vi "Material Theme Editor.vi"() -> ()   [LabVIEW 2021]
doc: "Convert existing material3 json files exported from Google to be used with TSC Material application VIs.\n\n<b>Code Developed By:</b>\nDaniel Coons\nTechnology Service Corporation\nwww.tsc.com/atcs"
uses:
  Material-Palette/Material-Palette.lvclass
  Material Theme/Material Theme.lvclass
  Material-Scheme/Material-Scheme.lvclass
  user32.dll
  <vilib>/Utility/traverseref.llb/VI Scripting - Traverse.lvlib
  <vilib>/Utility/traverseref.llb/TRef TravTarget.ctl
  Material-Scheme/View-User Colors.vi
  _theme-editor/Theme Config/Theme Config.lvclass
panel:
  in  "palette":bool
  in  "File Interaction":enum32{"convert--buton", "load--buton"}(radio)
  in  "tabs":enum32{"color", "palette", "json", "buttons"}(radio)
  in  "preview":bool
  in  "close":bool
  out "header":bool
  in  "save":bool
  in  "Theme Mode":u16(ring) items=["Light Theme", "Light Medium Contrast", "Light High Contrast", "Dark Theme", "Dark Medium Contrast", "Dark High Constrast"]
  in  "Tab Control":T1(tab)
  out "material JSON output":string
  in  "Color Level":u16(ring) items=["Primary", "Secondary", "Tertiary", "Error", "Primary Fixed", "Secondary Fixed", "Tertiary Fixed"]
  in  "Tab Control file":enum32{"convert", "load"}(tab)
  in  "LabVIEW material theme":path
  in  "json file path":path caption="Material Theme JSON File"
  # "Load a TSC Material Theme legacy XML file to see modes\nand palette colors and convert to JSON format for long-term\nsupport."
  # "Load a JSON M3 theme file from Google to \nview and edit the scheme."
  # "Can be generated through Figma or at:   https://material-foundation.github.io/material-theme-builder/<Material Website>"
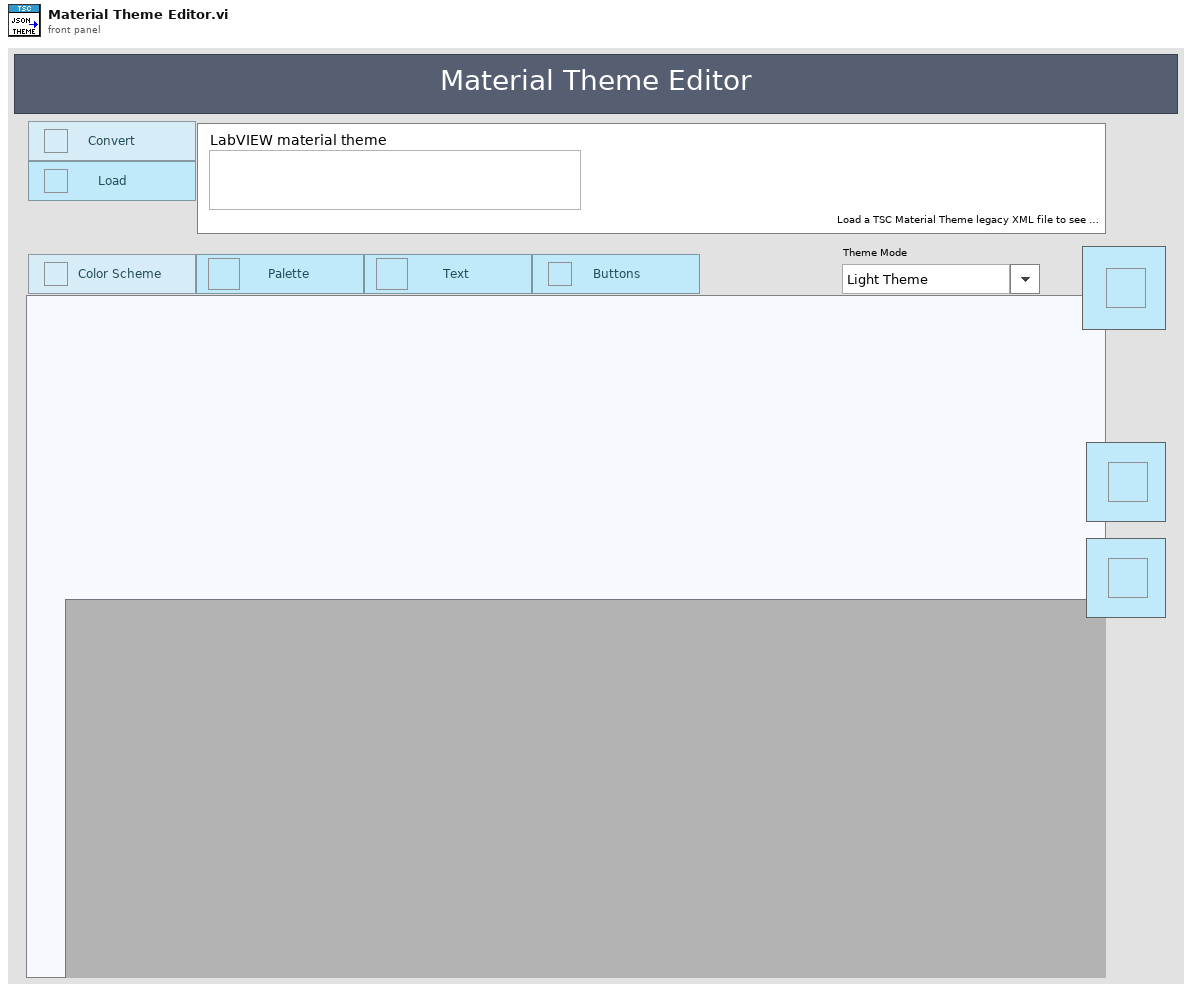
[diagram p1: front panel]
types:
  T1 = enum32{"Color Scheme", "Palette Variations", "JSON String", "buttons"}
  T2 = typedef "TRef TravTarget.ctl" = enum16{"FP", "BD", "Other"}
  T3 = enum16{"open", "replace", "create", "open or create", "replace or create", "replace or create with confirmation"}
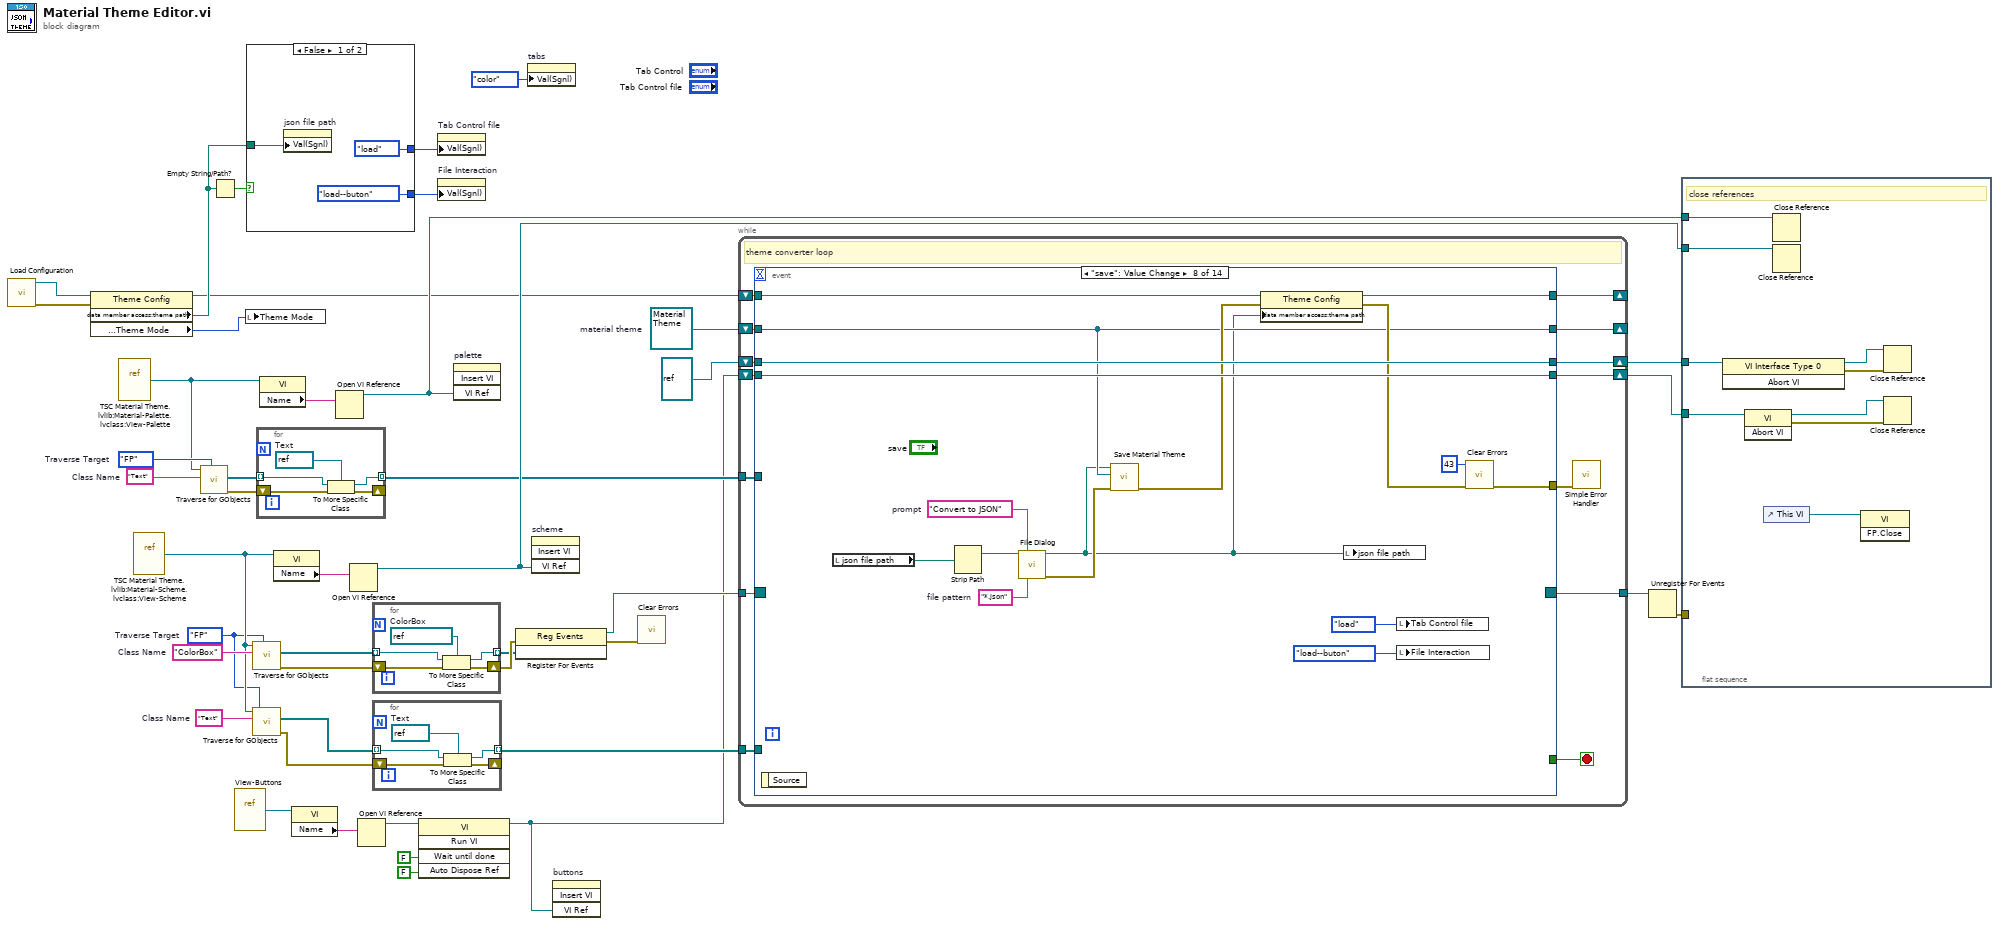
[diagram p0: block diagram]
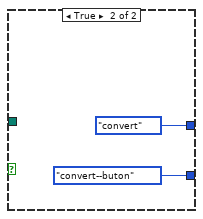
[diagram p2: hidden frame]
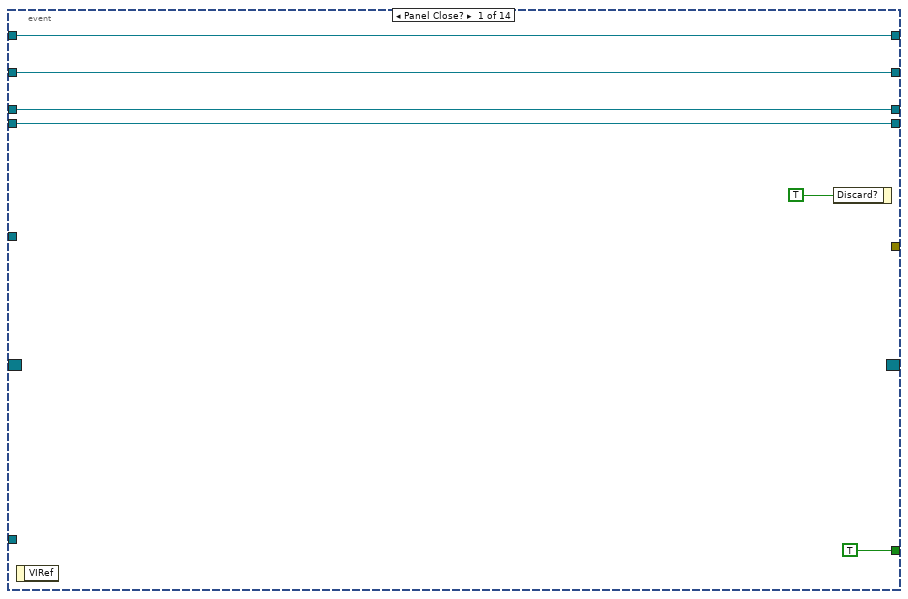
[diagram p3: hidden frame]
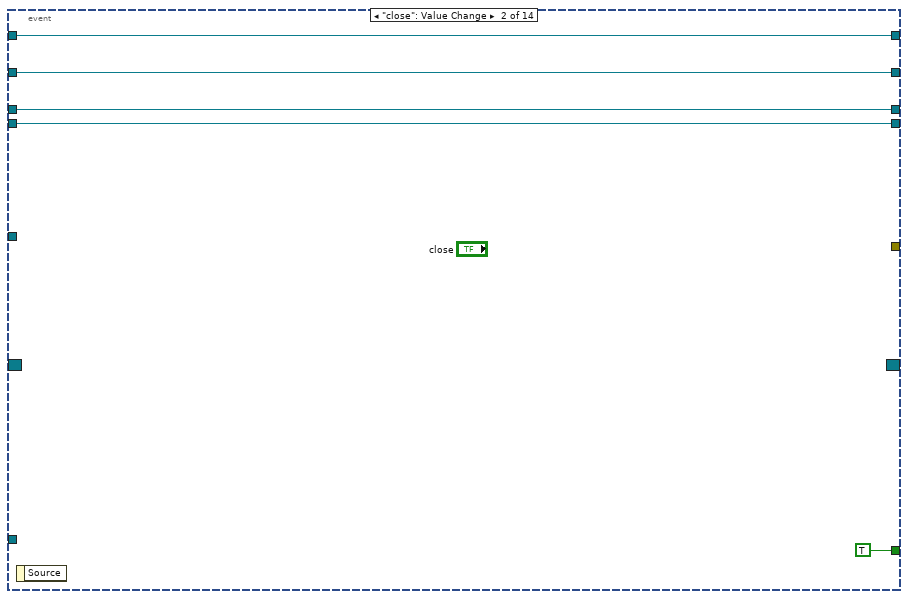
[diagram p4: hidden frame]
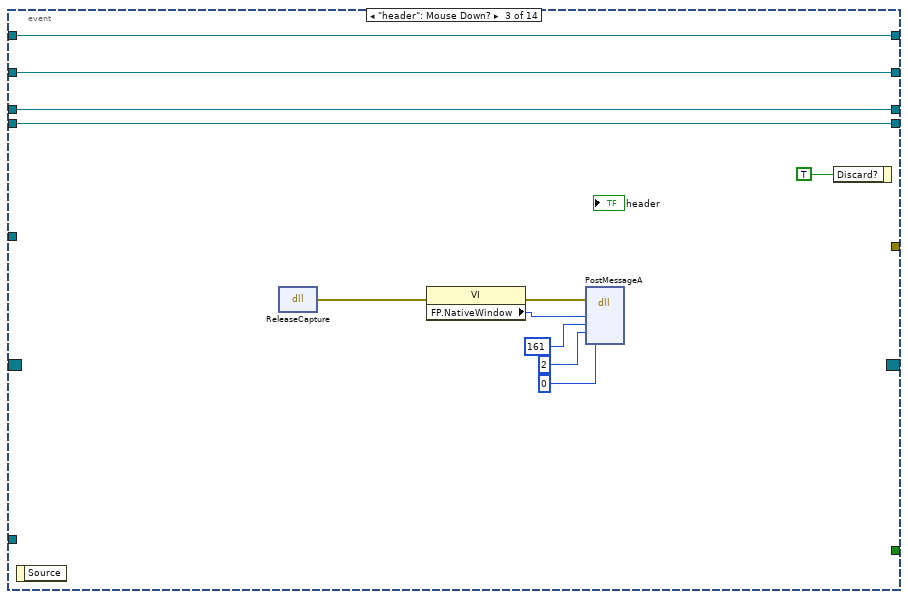
[diagram p5: hidden frame]
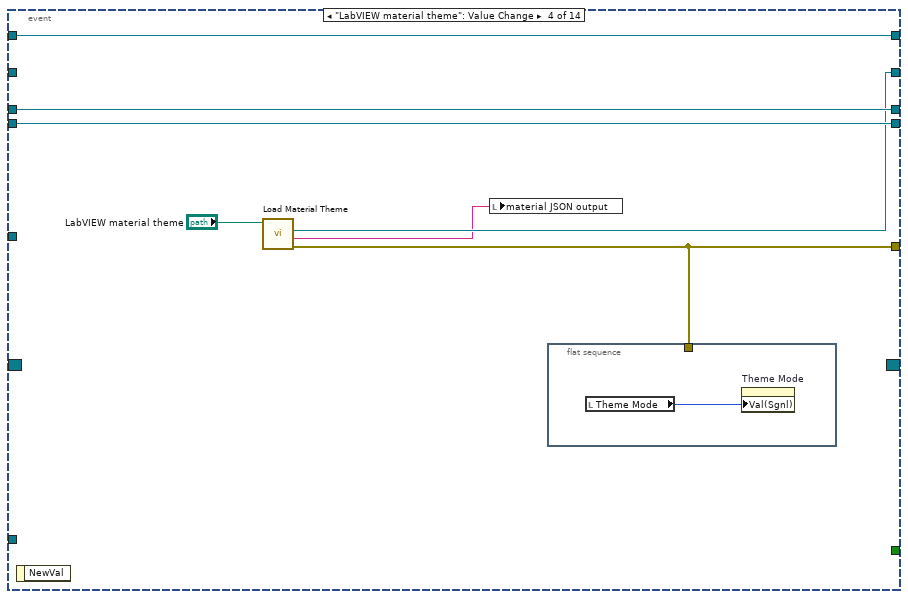
[diagram p6: hidden frame]
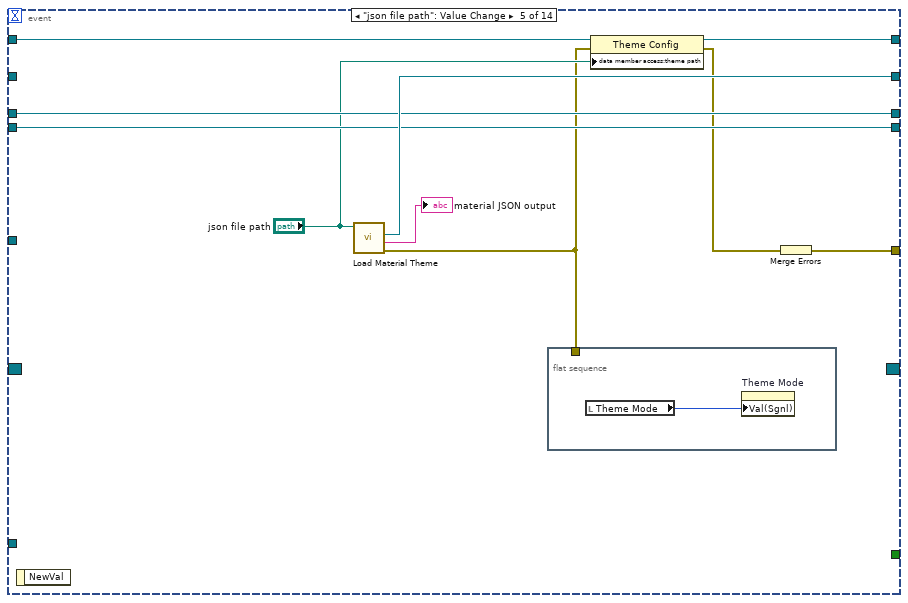
[diagram p7: hidden frame]
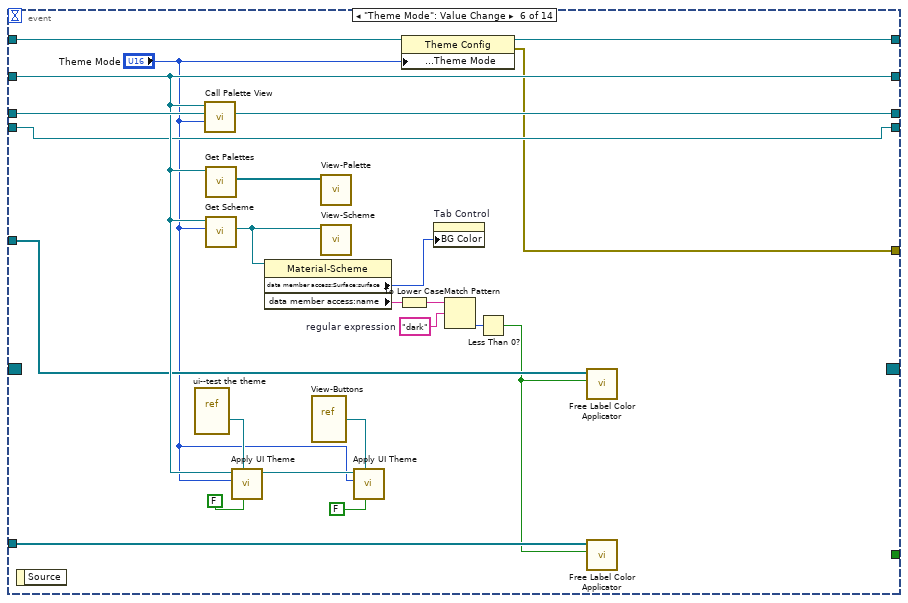
[diagram p8: hidden frame]
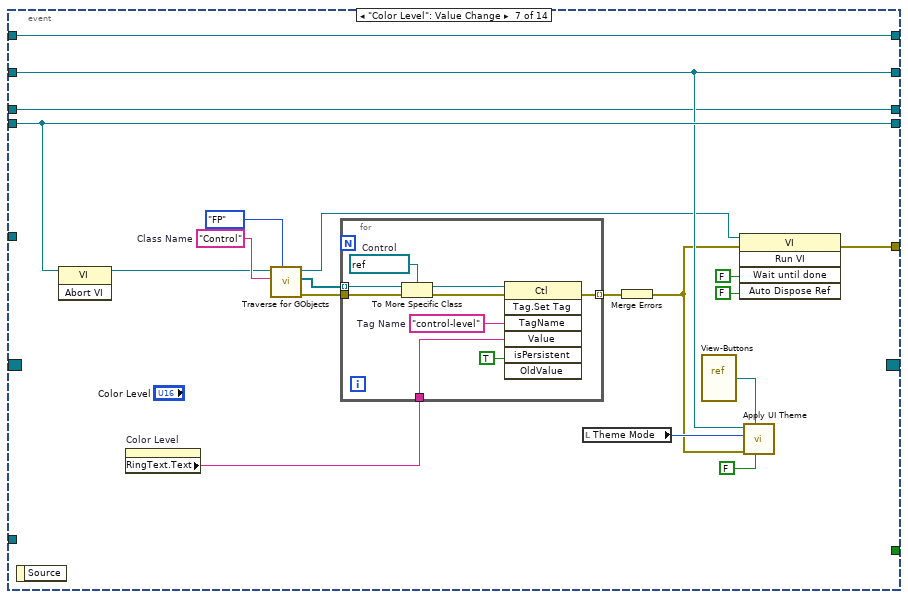
[diagram p9: hidden frame]
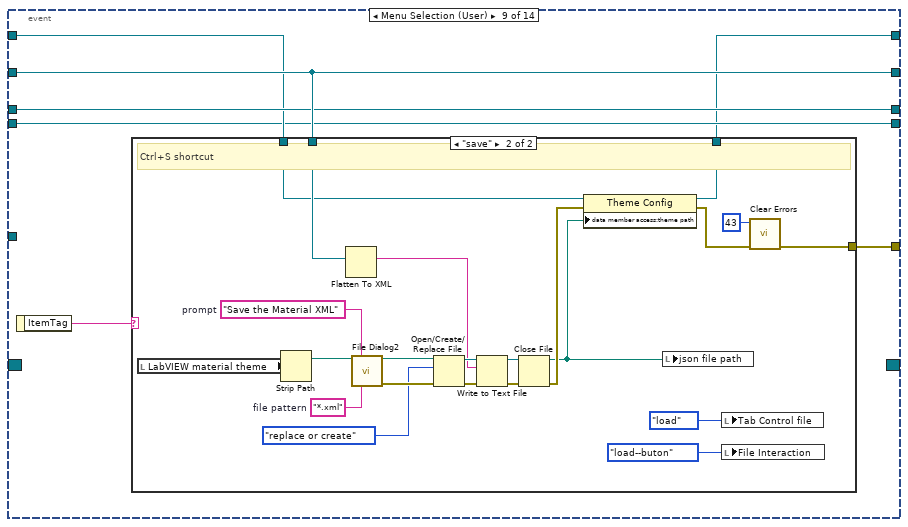
[diagram p10: hidden frame]
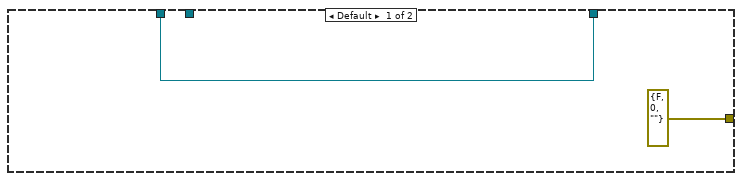
[diagram p11: hidden frame]
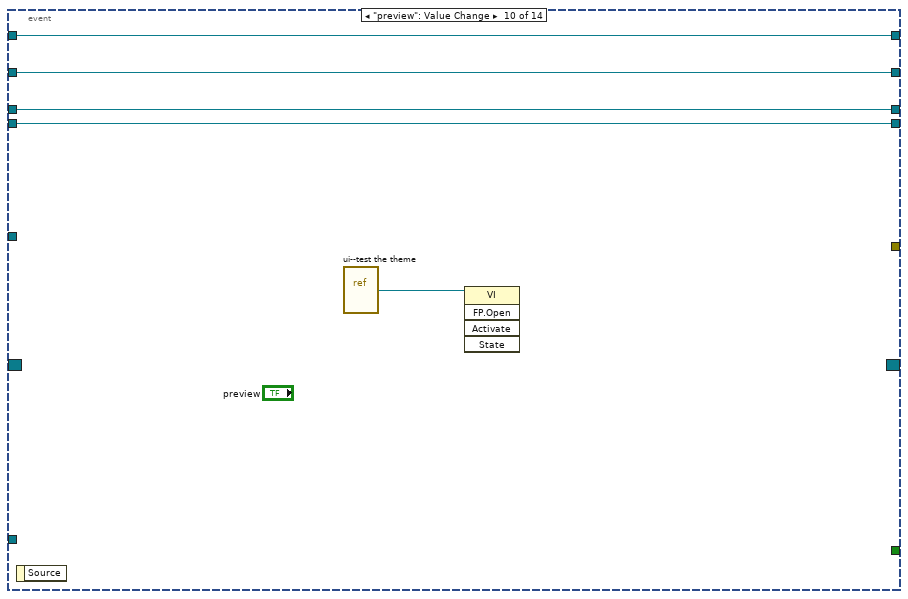
[diagram p12: hidden frame]
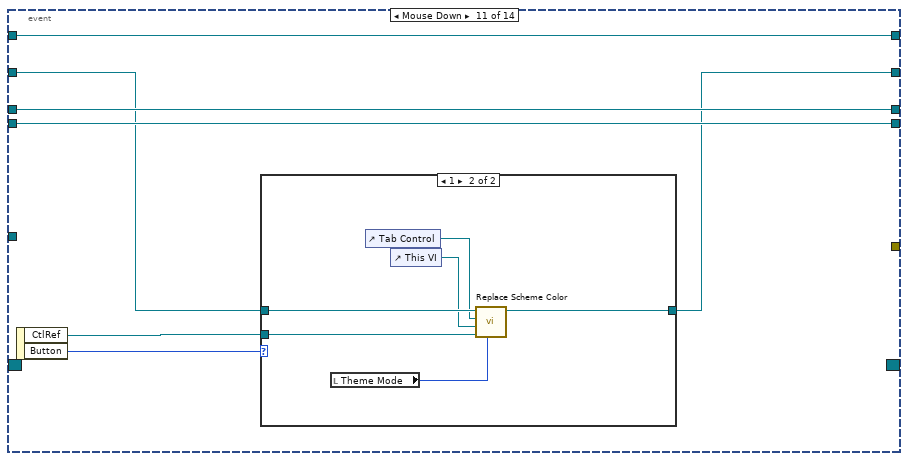
[diagram p13: hidden frame]
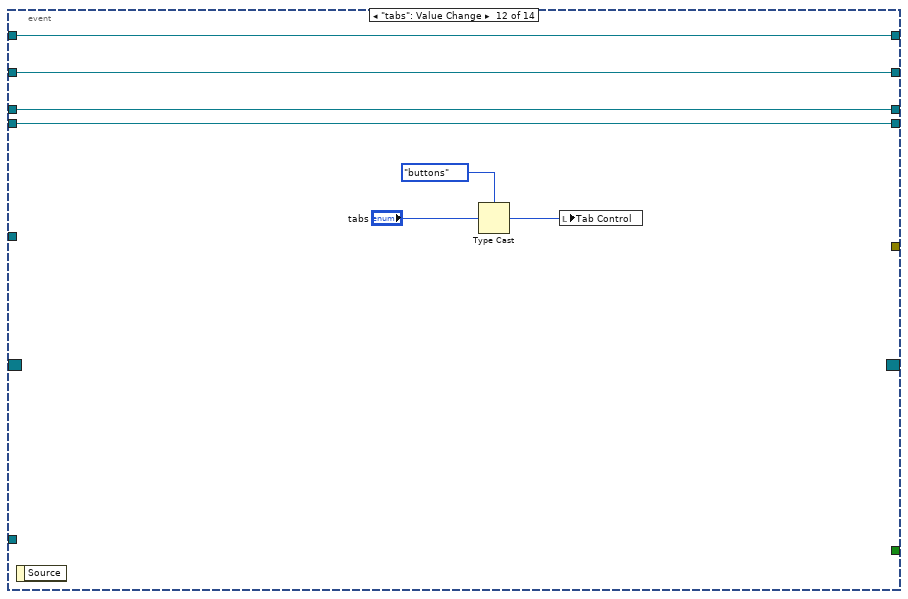
[diagram p15: hidden frame]
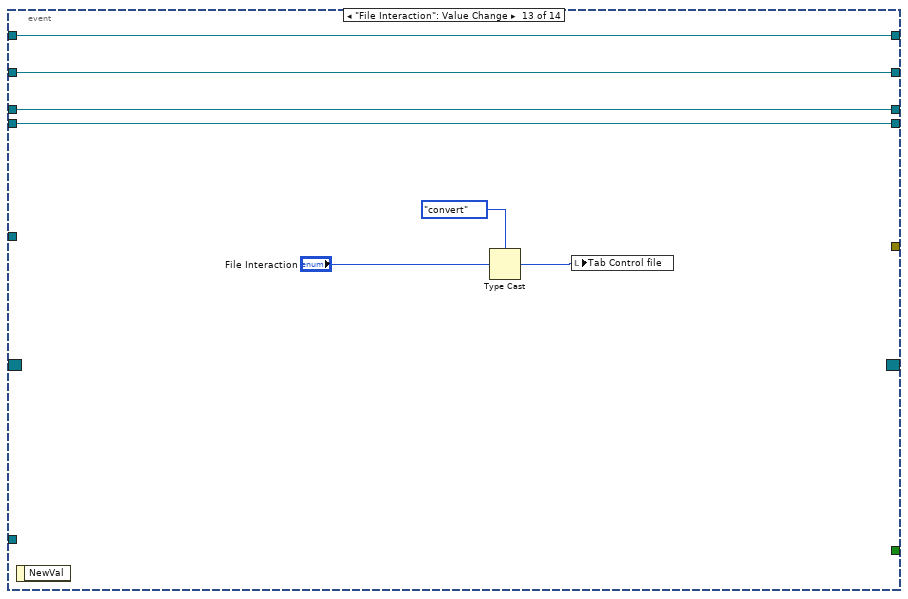
[diagram p16: hidden frame]
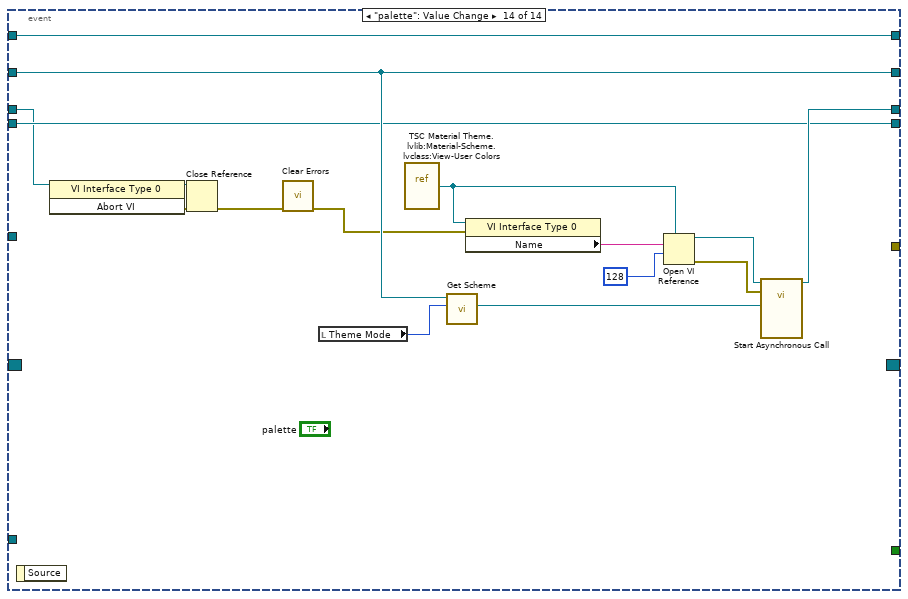
[diagram p17: hidden frame]
diagram:
  w24 = "Text"  # Class Name
  w27 = "Text"  # Class Name
  w28 = TRef_TravTarget."FP"  # Traverse Target
  w30 = refnum<class "Material Theme.lvclass"> refnum  # material theme
  w36 = "ColorBox"  # Class Name
  w22 = TRef_TravTarget."FP"  # Traverse Target
  n1 = call "Load Configuration.vi"() -> ("error out"=w10:errorcluster, "Theme Config out"=w9:refnum<class "Theme Config.lvclass">)  [unwired: 10 in]
  n2 = property class="Theme Config"(reference=w9, error in=w10) -> (reference out=w6:refnum<class "Theme Config.lvclass">, "data member access:theme path"=w8:path, "data member access:Theme Mode"=w3:u16)  [unwired: 1 out]
  n3 = vi-ref "TSC Material Theme.lvlib:Material-Palette.lvclass:View-Palette.vi"() -> (w7:refnum<vi>)
  n4 = vi-ref "TSC Material Theme.lvlib:Material-Scheme.lvclass:View-Scheme.vi"() -> (w23:refnum<vi>)
  n5 = call <vilib>:"Traverse for GObjects.vi"("Traverse Target"=w28, "Class Name"=w27, "VI Refnum"=w7) -> ("error out"=w41:errorcluster, "References"=w26:refnum<vi>[])  [unwired: 5 in, 2 out]
  n6 = Empty String/Path?(string/path=w8) -> (empty?=w29:bool)
  n7 = vi-ref "View-Buttons.vi"() -> (w17:refnum<vi>)
  n8 = local write "Theme Mode"(w3) -> ()
  n9 = case shown="False" w29 {
    tunnel: w8 -> [w47 _]
    tunnel: [enum32{"convert", "load"}."load" ("Value (Signaling)") enum32{"convert", "load"}."convert" ("Value (Signaling)")] -> w2
    tunnel: [enum32{"convert--buton", "load--buton"}."load--buton" ("Value (Signaling)") enum32{"convert--buton", "load--buton"}."convert--buton" ("Value (Signaling)")] -> w1
    frame False {
      n10 = property on="json file path" class="Path"("Val(Sgnl)"=w47) -> ()  [unwired: 2 in, 2 out]
    }
    frame True {
    }
  }
  n11 = call <vilib>:"Traverse for GObjects.vi"("Traverse Target"=w22, "Class Name"=w36, "VI Refnum"=w23) -> ("error out"=w44:errorcluster, "References"=w34:refnum<vi>[])  [unwired: 5 in, 2 out]
  n12 = call <vilib>:"Traverse for GObjects.vi"("Traverse Target"=w22, "Class Name"=w24, "VI Refnum"=w23) -> ("error out"=w40:errorcluster, "References"=w21:refnum<vi>[])  [unwired: 5 in, 2 out]
  n13 = for {
    tunnel: w26 -> [w51] mode=indexing
    shift-right: [w53] -> _
    shift-left: w41 -> [w54]
    tunnel: [w50] -> w25 mode=indexing
    w52 = refnum<vi> refnum  # Text
    n14 = To More Specific Class(target class=w52, reference=w51, error in=w54) -> (specific class reference=w50:refnum<vi>, error out=w53:errorcluster)
  }
  n15 = property class="VI"(reference=w7) -> ("Name"=w39:string)  [unwired: 1 in, 2 out]
  n16 = property class="VI"(reference=w23) -> ("Name"=w38:string)  [unwired: 1 in, 2 out]
  n17 = property class="VI"(reference=w17) -> ("Name"=w16:string)  [unwired: 1 in, 2 out]
  n18 = Open VI Reference(vi path=w39) -> (vi reference=w37:refnum<vi>)  [unwired: 5 in, 1 out]
  n19 = Open VI Reference(vi path=w38) -> (vi reference=w33:refnum<vi>)  [unwired: 5 in, 1 out]
  n20 = Open VI Reference(vi path=w16) -> (vi reference=w18:refnum<vi>)  [unwired: 5 in, 1 out]
  n21 = for {
    tunnel: w34 -> [w56] mode=indexing
    shift-right: [w58] -> w43
    shift-left: w44 -> [w59]
    tunnel: [w55] -> w32 mode=indexing
    w57 = refnum<vi> refnum  # ColorBox
    n22 = To More Specific Class(target class=w57, reference=w56, error in=w59) -> (specific class reference=w55:refnum<vi>, error out=w58:errorcluster)
  }
  n23 = for {
    tunnel: w21 -> [w61] mode=indexing
    shift-right: [w63] -> _
    shift-left: w40 -> [w64]
    tunnel: [w60] -> w20 mode=indexing
    w62 = refnum<vi> refnum  # Text
    n24 = To More Specific Class(target class=w62, reference=w61, error in=w64) -> (specific class reference=w60:refnum<vi>, error out=w63:errorcluster)
  }
  n25 = invoke class="VI" method="Run VI"(reference=w18, "Wait until done"=FALSE ("Wait Until Done"), "Auto Dispose Ref"=FALSE ("Auto Dispose Reference")) -> (reference out=w13:refnum<vi>)  [unwired: 2 in, 4 out]
  n26 = property on="Tab Control file" class="TabCtl (strict)"("Val(Sgnl)"=w2) -> ()  [unwired: 2 in, 2 out]
  n27 = property on="File Interaction" class="RadioBtnsControl (strict)"("Val(Sgnl)"=w1) -> ()  [unwired: 2 in, 2 out]
  n28 = invoke on="palette" class="SubPnl" method="Insert VI"("VI Ref"=w37) -> ()  [unwired: 3 in, 4 out]
  n29 = register-events(error in=w43, w32) -> (reference out=w35:refnum<event-registration>, error out=w42:errorcluster)  [unwired: 1 in]
  n30 = property on="tabs" class="RadioBtnsControl (strict)"("Val(Sgnl)"=enum32{"color", "palette", "json", "buttons"}."color" ("Value (Signaling)")) -> ()  [unwired: 2 in, 2 out]
  n31 = invoke on="scheme" class="SubPnl" method="Insert VI"("VI Ref"=w33) -> ()  [unwired: 3 in, 4 out]
  n32 = invoke on="buttons" class="SubPnl" method="Insert VI"("VI Ref"=w13) -> ()  [unwired: 3 in, 4 out]
  n33 = call <vilib>:"Clear Errors.vi"("error in (no error)"=w42) -> ()  [unwired: 5 in, 2 out]
  n34 = while {
    shift-right: [w76] -> _
    shift-left: w30 -> [w75]
    tunnel: w35 -> [w74]
    tunnel: [w73] -> w31
    tunnel: w25 -> [w72]
    tunnel: w20 -> [w71]
    shift-right: [w69] -> w12
    shift-left: refnum<vi> refnum -> [w68]
    shift-right: [w66] -> _
    shift-left: w6 -> [w67]
    shift-right: [w65] -> w4
    shift-left: w13 -> [w70]
    stop <- w77 stop-if-true
    # "theme converter loop"
    n35 = event shown="[7] \"save\": Value Change" {
      selector: w74 -> [_ _ _ _ _ _ _ _ _ _ _ _ _ _]
      dyn-events: [_ _ _ _ _ _ _ _ _ _ _ _ _ _] -> w73
      timeout: _ -> [_ _ _ _ _ _ _ _ _ _ _ _ _ _]
      tunnel: [TRUE TRUE _ _ _ _ _ _ _ _ _ _ _ _] -> w77
      tunnel: [w82 w89 w93 w102 w117 w129 w148 w172 w193 w223 w224 w244 w248 w267] -> w76
      tunnel: w75 -> [w82 w89 w93 _ _ w129 w148 w172 w193 w223 w225 w244 w248 w267]
      tunnel: [_ _ _ w103 w118 w120 w154 w175 w194 _ _ _ _ _] -> w78
      tunnel: w72 -> [_ _ _ _ _ w124 _ _ _ _ _ _ _ _]
      tunnel: w71 -> [_ _ _ _ _ w133 _ _ _ _ _ _ _ _]
      tunnel: w70 -> [w79 w85 w90 w105 w114 w125 w159 w177 w189 w219 w227 w238 w245 w257]
      tunnel: [w81 w87 w92 w107 w116 w128 w144 w182 w191 w221 w229 w240 w247 w259] -> w69
      tunnel: w68 -> [w81 w87 w92 w107 w116 w130 w144 w182 w191 w221 w229 w240 w247 w254]
      tunnel: w67 -> [w80 w86 w91 w106 w115 w126 w143 w179 w190 w220 w228 w239 w246 w258]
      tunnel: [w80 w86 w91 w106 w113 w122 w143 w178 w188 w220 w228 w239 w246 w258] -> w66
      tunnel: [w79 w85 w90 w105 w114 w125 w159 w177 w189 w219 w227 w238 w245 w257] -> w65
      event Panel Close? {
        n36 = event-data() -> ()  [unwired: 1 in, 1 out]
        n37 = event-data("Discard?"=TRUE) -> ()  [unwired: 1 in, 1 out]
      }
      event "close": Value Change {
        n38 = event-data() -> ()  [unwired: 1 in, 1 out]
      }
      event "header": Mouse Down? {
        n39 = event-data() -> ()  [unwired: 1 in, 1 out]
        n40 = dll-call lib="user32.dll" fn="ReleaseCapture"() -> (error out=w100:errorcluster)  [unwired: 4 in, 1 out]
        n41 = property class="VI"(error in=w100) -> (error out=w99:errorcluster, "FP.NativeWindow"=w94:u64)  [unwired: 1 in, 1 out]
        n42 = dll-call lib="user32.dll" fn="PostMessageA"(error in=w99, "hWnd"=w94, "Msg"=161, "wParam"=2, "lParam"=0) -> ()  [unwired: 7 in, 2 out]
        n43 = event-data("Discard?"=TRUE) -> ()  [unwired: 1 in, 1 out]
      }
      event "LabVIEW material theme": Value Change {
        n44 = event-data() -> ()  [unwired: 1 in, 1 out]
        n45 = call "Load Material Theme.vi"("file path"="LabVIEW material theme") -> ("error out"=w103:errorcluster, "text"=w101:string, "Theme"=w102:refnum<class "Material Theme.lvclass">)  [unwired: 8 in]
        n46 = local write "material JSON output"(w101) -> ()
        n47 = flat-sequence {
          tunnel: w103 -> [_]
          frame #0 {
            n48 = local read "Theme Mode"() -> (w108:u16)
            n49 = property on="Theme Mode" class="Ring (strict)"("Val(Sgnl)"=w108) -> ()  [unwired: 2 in, 2 out]
          }
        }
      }
      event "json file path": Value Change {
        n50 = event-data() -> ()  [unwired: 1 in, 1 out]
        n51 = call "Load Material Theme.vi"("file path"="json file path") -> ("error out"=w111:errorcluster, "text"=→"material JSON output":string, "Theme"=w117:refnum<class "Material Theme.lvclass">)  [unwired: 8 in]
        n52 = flat-sequence {
          tunnel: w111 -> [_]
          frame #0 {
            n53 = local read "Theme Mode"() -> (w119:u16)
            n54 = property on="Theme Mode" class="Ring (strict)"("Val(Sgnl)"=w119) -> ()  [unwired: 2 in, 2 out]
          }
        }
        n55 = property class="Theme Config"(reference=w115, error in=w111, "data member access:theme path"="json file path") -> (reference out=w113:refnum<class "Theme Config.lvclass">, error out=w110:errorcluster)
        n56 = Merge Errors(w110) -> (w118:errorcluster)
      }
      event "Theme Mode": Value Change {
        w136 = "dark"  # regular expression
        n57 = event-data() -> ()  [unwired: 1 in, 1 out]
        n58 = vi-ref "ui--test the theme.vi"() -> (w141:refnum<vi>)
        n59 = call "Call Palette View.vi"("Theme Mode"="Theme Mode", "VI ref in"=w130, "Material Theme"=w129) -> ("VI ref"=w128:refnum<vi>)  [unwired: 7 in, 1 out]
        n60 = call "Get Palettes.vi"("Material Theme in"=w129) -> ("Material-Palettes"=w142:refnum<class "Material-Palette.lvclass">[])  [unwired: 8 in, 2 out]
        n61 = call "Get Scheme.vi"("Theme"="Theme Mode", "Material Theme in"=w129) -> ("Material-Scheme"=w139:refnum<class "Material-Scheme.lvclass">)  [unwired: 7 in, 2 out]
        n62 = call "Apply UI Theme.vi"("save?"=FALSE, "VI Refnum"=w141, "Theme Mode"="Theme Mode", "Material Theme in"=w129) -> ("Material Theme out"=w127:refnum<class "Material Theme.lvclass">)  [unwired: 6 in, 1 out]
        n63 = property class="Material-Scheme"(reference=w139) -> ("data member access:Surface:surface"=w138:u32, "data member access:name"=w137:string)  [unwired: 1 in, 2 out]
        n64 = vi-ref "View-Buttons.vi"() -> (w131:refnum<vi>)
        n65 = call "View-Palette.vi"("Array"=w142) -> ()  [unwired: 11 in]
        n66 = call "View-Scheme.vi"("Material-Scheme.lvclass"=w139) -> ()  [unwired: 11 in]
        n67 = call "Apply UI Theme.vi"("save?"=FALSE, "VI Refnum"=w131, "Theme Mode"="Theme Mode", "Material Theme in"=w127) -> ()  [unwired: 6 in, 2 out]
        n68 = To Lower Case(string=w137) -> (all lower case string=w135:string)
        n69 = property class="Theme Config"(reference=w126, "data member access:Theme Mode"="Theme Mode") -> (reference out=w122:refnum<class "Theme Config.lvclass">, error out=w120:errorcluster)  [unwired: 1 in]
        n70 = property on="Tab Control" class="TabCtl (strict)"("BG Color"=w138) -> ()  [unwired: 2 in, 2 out]
        n71 = Match Pattern(string=w135, regular expression=w136) -> (offset past match=w134:i32)  [unwired: 1 in, 3 out]
        n72 = Less Than 0?(x=w134) -> (x < 0?=w123:bool)
        n73 = call "Free Label Color Applicator.vi"("Dark Text?"=w123, "Text Labels"=w124) -> ()  [unwired: 10 in]
        n74 = call "Free Label Color Applicator.vi"("Dark Text?"=w123, "Text Labels"=w133) -> ()  [unwired: 10 in]
      }
      event "Color Level": Value Change {
        w161 = "Control"  # Class Name
        n75 = event-data() -> ()  [unwired: 1 in, 1 out]
        n76 = invoke class="VI" method="Abort VI"(reference=w159) -> (reference out=w153:refnum<vi>)  [unwired: 2 in, 2 out]
        n77 = property on="Color Level" class="Ring (strict)"() -> ("RingText.Text"=w156:string)  [unwired: 2 in, 2 out]
        n78 = call <vilib>:"Traverse for GObjects.vi"("Traverse Target"=TRef_TravTarget."FP", "Class Name"=w161, "VI Refnum"=w153) -> ("error out"=w157:errorcluster, "References"=w158:refnum<vi>[], "dup VI Refnum"=w145:refnum<vi>)  [unwired: 5 in, 1 out]
        n79 = for {
          tunnel: w158 -> [w169] mode=indexing
          tunnel: w157 -> [w168]
          tunnel: w156 -> [w164]
          tunnel: [w162] -> w155 mode=indexing
          w167 = refnum<vi> refnum  # Control
          w170 = "control-level"  # Tag Name
          n80 = To More Specific Class(target class=w167, reference=w169, error in=w168) -> (specific class reference=w165:refnum<vi>, error out=w166:errorcluster)
          n81 = invoke class="Ctl" method="Tag.Set Tag"(reference=w165, error in=w166, "TagName"=w170, "Value"=w164, "isPersistent"=TRUE ("Is Persistent?")) -> (error out=w162:errorcluster)  [unwired: 2 in, 6 out]
        }
        n82 = local read "Theme Mode"() -> (w147:u16)
        n83 = Merge Errors(w155) -> (w146:errorcluster)
        n84 = vi-ref "View-Buttons.vi"() -> (w150:refnum<vi>)
        n85 = invoke class="VI" method="Run VI"(reference=w145, error in=w146, "Wait until done"=FALSE ("Wait Until Done"), "Auto Dispose Ref"=FALSE ("Auto Dispose Reference")) -> (error out=w154:errorcluster)  [unwired: 1 in, 4 out]
        n86 = call "Apply UI Theme.vi"("save?"=FALSE, "VI Refnum"=w150, "error in"=w146, "Theme Mode"=w147, "Material Theme in"=w148) -> ()  [unwired: 5 in, 2 out]
      }
      event "save": Value Change {
        w183 = "Convert to JSON"  # prompt
        w186 = "*.json"  # file pattern
        n87 = event-data() -> ()  [unwired: 1 in, 1 out]
        n88 = local read "json file path"() -> (w185:path)
        n89 = Strip Path(path=w185) -> (stripped path=w184:path)  [unwired: 1 out]
        n90 = call "File Dialog"("start path"=w184, "prompt"=w183, "pattern (all files)"=w186) -> ("selected path"=w171:path, "error out"=w174:errorcluster)  [unwired: 9 in, 2 out]
        n91 = call "Save Material Theme.vi"("error in"=w174, "Theme"=w172, "file path"=w171) -> ("error out"=w173:errorcluster)  [unwired: 7 in, 1 out]
        n92 = property class="Theme Config"(reference=w179, error in=w173, "data member access:theme path"=w171) -> (reference out=w178:refnum<class "Theme Config.lvclass">, error out=w176:errorcluster)
        n93 = local write "json file path"(w171) -> ()
        n94 = local write "Tab Control file"(enum32{"convert", "load"}."load" ("Tab Control file")) -> ()
        n95 = local write "File Interaction"(enum32{"convert--buton", "load--buton"}."load--buton" ("File Interaction")) -> ()
        n96 = call <vilib>:"Clear Errors.vi"("error in (no error)"=w176, "specific error code to clear (0: all)"=43) -> ("error out"=w175:errorcluster)  [unwired: 4 in, 1 out]
      }
      event Menu Selection (User) {
        n97 = event-data() -> ("ItemTag"=w192:string)  [unwired: 1 in]
        n98 = case shown="\"save\"" w192 {
          tunnel: w193 -> [_ w215]
          tunnel: [errorcluster {"status"=FALSE, "code"=0, "source"=""} ("error out") w197] -> w194
          tunnel: w190 -> [w195 w202]
          tunnel: [w195 w201] -> w188
          frame Default {
          }
          frame "save" {
            w208 = "Save the Material XML"  # prompt
            w207 = "*.xml"  # file pattern
            # "Ctrl+S shortcut"
            n99 = local read "LabVIEW material theme"() -> (w210:path)
            n100 = Strip Path(path=w210) -> (stripped path=w209:path)  [unwired: 1 out]
            n101 = Flatten To XML(6:w215) -> (2:w205:string)
            n102 = call "File Dialog2"("start path"=w209, "prompt"=w208, "pattern (all files)"=w207) -> ("selected path"=w211:path, "error out"=w216:errorcluster)  [unwired: 9 in, 2 out]
            n103 = Open/Create/Replace File(file path (use dialog)=w211, error in=w216, operation (0:open)=T3."replace or create") -> (refnum out=w213:refnum<file>, error out=w217:errorcluster)  [unwired: 3 in, 1 out]
            n104 = Write to Text File(file (use dialog)=w213, text=w205, error in=w217) -> (refnum out=w212:refnum<file>, error out=w218:errorcluster)  [unwired: 1 in, 1 out]
            n105 = Close File(refnum=w212, error in=w218) -> (path=w199:path, error out=w200:errorcluster)
            n106 = property class="Theme Config"(reference=w202, error in=w200, "data member access:theme path"=w199) -> (reference out=w201:refnum<class "Theme Config.lvclass">, error out=w198:errorcluster)
            n107 = local write "json file path"(w199) -> ()
            n108 = local write "Tab Control file"(enum32{"convert", "load"}."load" ("Tab Control file")) -> ()
            n109 = local write "File Interaction"(enum32{"convert--buton", "load--buton"}."load--buton" ("File Interaction")) -> ()
            n110 = call <vilib>:"Clear Errors.vi"("error in (no error)"=w198, "specific error code to clear (0: all)"=43) -> ("error out"=w197:errorcluster)  [unwired: 4 in, 1 out]
          }
        }
      }
      event "preview": Value Change {
        n111 = event-data() -> ()  [unwired: 1 in, 1 out]
        n112 = vi-ref "ui--test the theme.vi"() -> (w222:refnum<vi>)
        n113 = invoke class="VI" method="FP.Open"(reference=w222) -> ()  [unwired: 4 in, 5 out]
      }
      event Mouse Down {
        n114 = event-data() -> ("CtlRef"=w230:refnum<vi>, "Button"=w226:u16)  [unwired: 1 in]
        n115 = case shown="1" w226 {
          tunnel: w230 -> [_ w234]
          tunnel: w225 -> [w231 w237]
          tunnel: [w231 w236] -> w224
          frame 0, Default {
          }
          frame 1 {
            n116 = local read "Theme Mode"() -> (w235:u16)
            n117 = control-ref of="Tab Control"() -> (w233:refnum<vi>)
            n118 = control-ref of="This VI"() -> (w232:refnum<vi>)
            n119 = call "Replace Scheme Color.vi"("Theme Mode"=w235, "Colorbox ref in"=w234, "This VI"=w232, "TabControl in"=w233, "Material Theme in"=w237) -> ("Material Theme out"=w236:refnum<class "Material Theme.lvclass">)  [unwired: 6 in]
          }
        }
      }
      event "tabs": Value Change {
        n120 = event-data() -> ()  [unwired: 1 in, 1 out]
        n121 = Type Cast(type=T1."buttons" ("Tab Control"), x="tabs") -> (*(type *) &x=w241:T1)
        n122 = local write "Tab Control"(w241) -> ()
      }
      event "File Interaction": Value Change {
        n123 = event-data() -> ()  [unwired: 1 in, 1 out]
        n124 = Type Cast(type=enum32{"convert", "load"}."convert" ("Tab Control file"), x="File Interaction") -> (*(type *) &x=w250:enum32{"convert", "load"})
        n125 = local write "Tab Control file"(w250) -> ()
      }
      event "palette": Value Change {
        n126 = event-data() -> ()  [unwired: 1 in, 1 out]
        n127 = invoke class="VI Interface Type 0" method="Abort VI"(reference=w254) -> (reference out=w253:refnum<vi>, error out=w252:errorcluster)  [unwired: 2 in, 1 out]
        n128 = Close Reference(reference=w253, error in (no error)=w252) -> (error out=w256:errorcluster)
        n129 = call <vilib>:"Clear Errors.vi"("error in (no error)"=w256) -> ("error out"=w255:errorcluster)  [unwired: 5 in, 1 out]
        n130 = local read "Theme Mode"() -> (w266:u16)
        n131 = vi-ref "TSC Material Theme.lvlib:Material-Scheme.lvclass:View-User Colors.vi"() -> (w261:refnum<vi>)
        n132 = call "Get Scheme.vi"("Theme"=w266, "Material Theme in"=w267) -> ("Material-Scheme"=w265:refnum<class "Material-Scheme.lvclass">)  [unwired: 7 in, 2 out]
        n133 = property class="VI Interface Type 0"(reference=w261, error in=w255) -> ("Name"=w264:string)  [unwired: 2 out]
        n134 = Open VI Reference(type specifier VI Refnum (for type only)=w261, vi path=w264, options=128) -> (vi reference=w262:refnum<vi>, error out=w260:errorcluster)  [unwired: 3 in]
        n135 = call-by-ref "Start Asynchronous Call"(reference=w262, error in=w260, "Material-Scheme.lvclass"=w265) -> (reference out=w259:refnum<vi>)  [unwired: 11 in, 1 out]
      }
    }
    n136 = call <vilib>:"Simple Error Handler.vi"("error in (no error)"=w78) -> ()  [unwired: 4 in, 5 out]
  }
  n137 = Unregister For Events(event registration refnum=w31) -> (error out=w5:errorcluster)  [unwired: 1 in]
  n138 = flat-sequence {
    tunnel: w37 -> [w276]
    tunnel: w33 -> [w275]
    tunnel: w12 -> [w270]
    tunnel: w5 -> [_]
    tunnel: w4 -> [w269]
    frame #0 {
      # "close references"
      n139 = invoke class="VI Interface Type 0" method="Abort VI"(reference=w270) -> (reference out=w271:refnum<vi>, error out=w272:errorcluster)  [unwired: 2 in, 1 out]
      n140 = invoke class="VI" method="Abort VI"(reference=w269) -> (reference out=w274:refnum<vi>, error out=w273:errorcluster)  [unwired: 2 in, 1 out]
      n141 = control-ref of="This VI"() -> (w268:refnum<vi>)
      n142 = Close Reference(reference=w276) -> ()  [unwired: 1 in, 1 out]
      n143 = Close Reference(reference=w275) -> ()  [unwired: 1 in, 1 out]
      n144 = invoke class="VI" method="FP.Close"(reference=w268) -> ()  [unwired: 2 in, 3 out]
      n145 = Close Reference(reference=w271, error in (no error)=w272) -> ()  [unwired: 1 out]
      n146 = Close Reference(reference=w274, error in (no error)=w273) -> ()  [unwired: 1 out]
    }
  }
